vi "rtlsdr_open.vi"(8 "error in":errorcluster, 9 "number of tries to connect":i32=5, 10 "remote port":u16=1234, 11 "address":string="127.0.0.1") -> (0 "error out":errorcluster, 3 "ref":refnum<k5>)   [LabVIEW 2011]
panel:
  # "Outputs:"
  # "Inputs:"
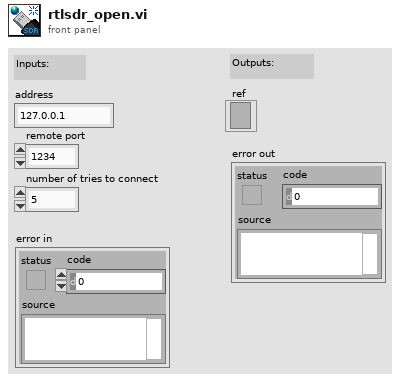
[diagram p1: front panel]
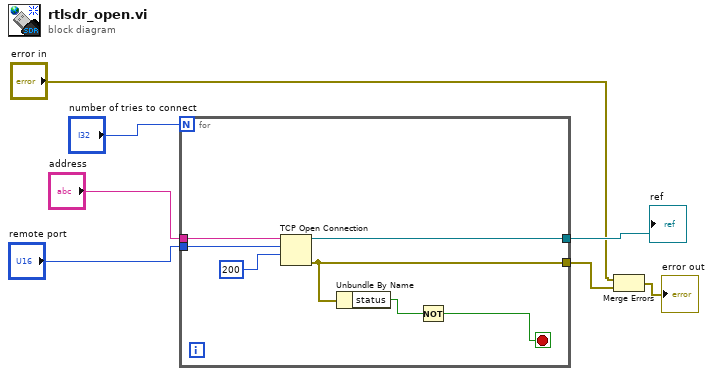
[diagram p0: block diagram]
diagram:
  n1 = for {
    N: "number of tries to connect" -> [_]
    tunnel: "address" -> [w14]
    tunnel: "remote port" -> [w13]
    tunnel: [w9] -> w2
    tunnel: [w8] -> w4
    stop <- w10 stop-if-true
    n2 = TCP Open Connection(address=w14, remote port or service name=w13, timeout ms (60000)=200) -> (connection ID=w8:refnum<k5>, error out=w9:errorcluster)  [unwired: 2 in]
    n3 = Unbundle By Name(w9) -> ("status"=w11:bool)
    n4 = Not(x=w11) -> (.not. x?=w10:bool)
  }
  "ref" <- w4
  n5 = Merge Errors("error in", w2) -> (→"error out":errorcluster)
